vi "DCA Compute Pi-R3.vi"(1 "Measurement Values":T1) -> (0 "Pi-R3":dbl)   [LabVIEW 2011]
uses:
  TypeDefs/DCA Measurement Values.ctl
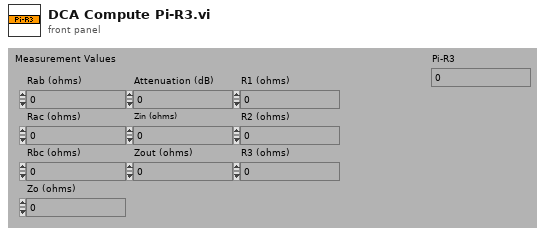
[diagram p1: front panel]
types:
  T1 = typedef "DCA Measurement Values.ctl" = cluster{"Rab (ohms)":dbl, "Rac (ohms)":dbl, "Rbc (ohms)":dbl, "Zo (ohms)":dbl, "Attenuation (dB)":dbl, "Zin (ohms)":dbl, "Zout (ohms)":dbl, "R1 (ohms)":dbl, "R2 (ohms)":dbl, "R3 (ohms)":dbl}
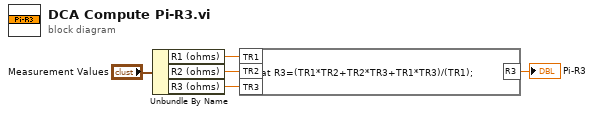
[diagram p0: block diagram]
diagram:
  n1 = Unbundle By Name("Measurement Values") -> ("R1 (ohms)"=w4:dbl, "R2 (ohms)"=w3:dbl, "R3 (ohms)"=w2:dbl)
  n2 = formula code="float R3=(TR1*TR2+TR2*TR3+TR1*TR3)/(TR1);"("TR1"=w4, "TR2"=w3, "TR3"=w2) -> ("R3"=→"Pi-R3":dbl)
